vi "SVL Decimated Exp Avg Sound Level (N Ch).vi"(6 "restart averaging (F)":bool, 7 "decimation factor":i32=-1, 8 "error in (no error)":errorcluster, 9 "time constant [ms]":dbl=125.0 format="%.2f", 10 "exponential mode":enum16{"Slow", "Fast", "Impulse", "Custom"}(ring)=enum."Fast", 11 "scaled signals [EU]":waveform(dbl)[](array[waveform])) -> (0 "error out":errorcluster, 1 "actual time constant [ms]":dbl=nan format="%.2f", 2 "unit labels":string[](array[string]), 3 "decimated exp avg sound levels [dB EU]":waveform(dbl)[](array[waveform]), 5 "actual decimation factor":i32=-1)   [LabVIEW 2017, in "SoundVib_SoundLevel.lvlib"]
doc: "Computes the exponential averaged sound level of <B>scaled signal [EU]</B> of <B>exponential mode</B> and decimates this sound level by <B>decimation factor</B>. <B>scaled signal [EU]</B> should have a zero DC component. You can attenuate the DC component with hardware AC-coupling filters and with software high-pass filters. Wire data to the <B>scaled signal [EU]</B> input to determine the polymorphic instance to use or manually select the instance."
uses:
  <vilib>/addons/Sound and Vibration/svt_Level/SoundVib_SoundLevel.lvlib
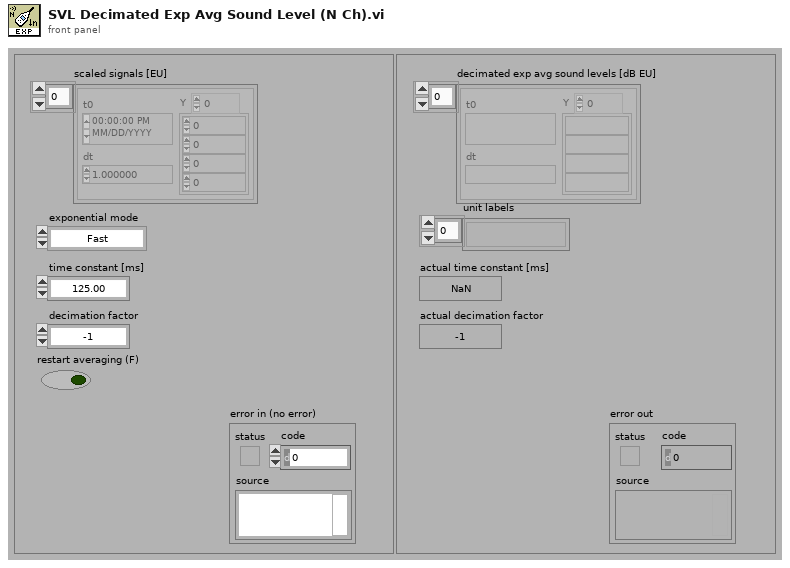
[diagram p1: front panel]
types:
  T1 = enum16{"RMS", "Running RMS", "Exp avg  ", "Dec exp avg ", "Peak", "Crest"}
  T2 = enum16{"Reset filter", "Restart averaging", "Continue processing"}
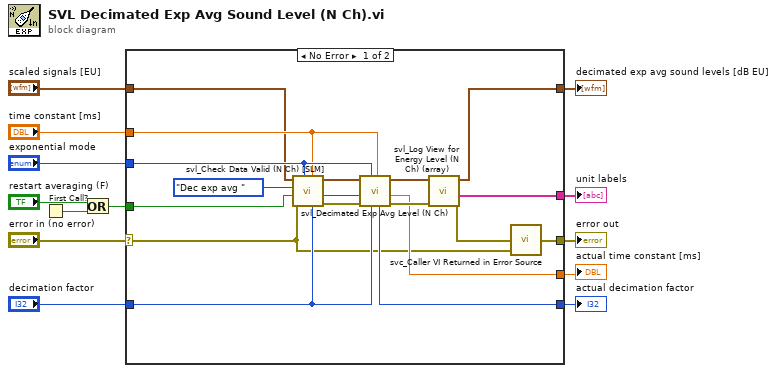
[diagram p0: block diagram]
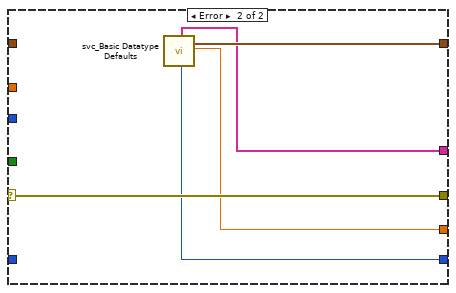
[diagram p2: hidden frame]
diagram:
  n1 = First Call?() -> (First Call?: T/F=w9:bool)
  n2 = Or(x="restart averaging (F)", y=w9) -> (x .or. y?=w8:bool)
  n3 = case shown="No Error" "error in (no error)" {
    selector: "error in (no error)" -> [w14 w36]
    tunnel: "scaled signals [EU]" -> [w17 _]
    tunnel: [w23 w36] -> w12
    tunnel: [w27 w34] -> w11
    tunnel: w8 -> [w22 _]
    tunnel: [w16 w35] -> w7
    tunnel: "exponential mode" -> [w26 _]
    tunnel: "decimation factor" -> [w20 _]
    tunnel: [w25 w33] -> w4
    tunnel: "time constant [ms]" -> [w19 _]
    tunnel: [w24 w32] -> w2
    frame No Error {
      n4 = call <vilib>:"svl_Check Data Valid (N Ch) [SLM].vi"("decimation factor"=w20, "time constant [ms]"=w19, "exponential mode"=w26, "error in (no error)"=w14, "restart averaging (F)"=w22, "level analysis"=T1."Dec exp avg " ("Level Analysis"), "scaled signals [EU]"=w17) -> ("error out"=w31:errorcluster, "processing state"=w21:T2, "dup scaled signals [EU]"=w15:waveform(dbl)[])  [unwired: 2 in]
      n5 = call <vilib>:"svl_Decimated Exp Avg Level (N Ch).vi"("time constant"=w19, "decimation factor"=w20, "exponential mode"=w26, "error in (no error)"=w31, "processing state"=w21, "scaled signals"=w15) -> ("error out"=w30:errorcluster, "actual time constant [ms]"=w24:dbl, "scaled signals"=w29:waveform(dbl)[], "actual decimation factor"=w25:i32)  [unwired: 2 in]
      n6 = call <vilib>:"svl_Log View for Energy Level (N Ch) (array).vi"("error in (no error)"=w30, "scaled signals"=w29) -> ("error out"=w28:errorcluster, "unit labels"=w27:string[], "scaled signals"=w16:waveform(dbl)[])  [unwired: 7 in]
      n7 = call <vilib>:"svc_Caller VI Returned in Error Source.vi"("warning input to caller"=w14, "error in (no error)"=w28) -> ("error out"=w23:errorcluster)  [unwired: 3 in]
    }
    frame Error {
      n8 = call <vilib>:"svc_Basic Datatype Defaults.vi"() -> ("empty array of strings"=w34:string[], "zero I32"=w33:i32, "empty array of waveforms"=w35:waveform(dbl)[], "NaN"=w32:dbl)  [unwired: 7 in, 9 out]
    }
  }
  "decimated exp avg sound levels [dB EU]" <- w7
  "actual time constant [ms]" <- w2
  "unit labels" <- w11
  "error out" <- w12
  "actual decimation factor" <- w4
